vi "insertXMLNode.vi"(8 "error in (no error)":errorcluster, 9 "createInNodePath":string, 10 "xmlNodeString":string, 11 "SettingsManager in":refnum<class "SettingsManager.lvclass">) -> (0 "error out":errorcluster, 3 "SettingsManager out":refnum<class "SettingsManager.lvclass">)   [LabVIEW 2009, in "Tools.lvlib" / "Settings.lvlib" / "SettingsManager.lvclass"]
uses:
  SettingsManager.lvclass
  SettingsManager.lvclass/SettingsManager.ctl
  xmlNode/xmlNode.lvclass
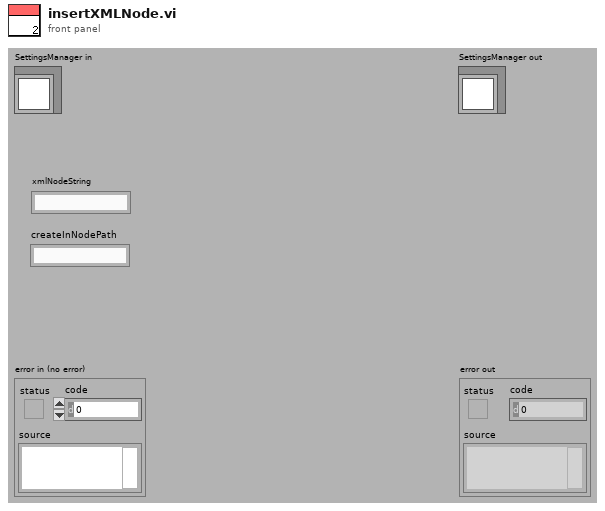
[diagram p1: front panel]
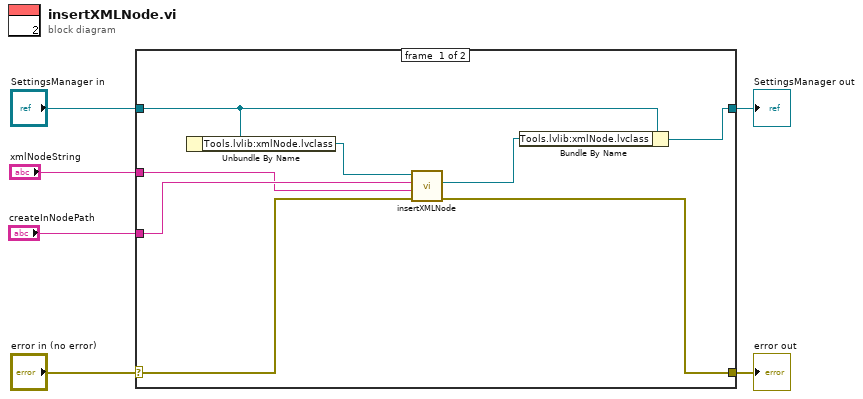
[diagram p0: block diagram]
diagram:
  n1 = case shown="No Error" "error in (no error)" {
    selector: "error in (no error)" -> [w10 w16]
    tunnel: [w9 w16] -> w5
    tunnel: [w12 w15] -> w3
    tunnel: "SettingsManager in" -> [w13 w15]
    tunnel: "xmlNodeString" -> [w7 _]
    tunnel: "createInNodePath" -> [w8 _]
    frame #0 {
      n2 = Unbundle By Name(w13) -> ("Tools.lvlib:xmlNode.lvclass"=w14:refnum<class "xmlNode.lvclass">)
      n3 = call-dynamic "insertXMLNode.vi"("error in (no error)"=w10, "xmlString"=w7, "xmlPath"=w8, "xmlNode in"=w14) -> ("error out"=w9:errorcluster, "newXMLNode"=w11:refnum<class "xmlNode.lvclass">)  [unwired: 5 in, 1 out]
      n4 = Bundle By Name(cluster=w13, "Tools.lvlib:xmlNode.lvclass"=w11) -> (w12:refnum<class "SettingsManager.lvclass">)
    }
    frame #1 {
    }
  }
  "error out" <- w5
  "SettingsManager out" <- w3
